vi "Default Cfg File Path.vi"(8 "error in (no error)":errorcluster) -> (0 "error out":errorcluster, 3 "Default Path":path)   [LabVIEW 2018]
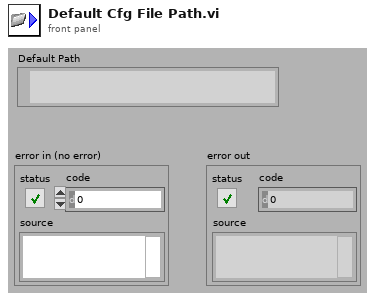
[diagram p1: front panel]
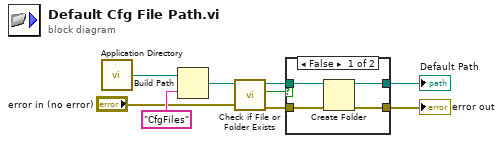
[diagram p0: block diagram]
diagram:
  n1 = call <vilib>:"Application Directory.vi"() -> ("Application Directory"=w8:path)
  n2 = Build Path(base path=w8, name or relative path="CfgFiles") -> (appended path=w4:path)
  n3 = call <vilib>:"Check if File or Folder Exists.vi"("error in (no error)"="error in (no error)", "path"=w4) -> ("error out"=w5:errorcluster, "file or folder exists?"=w6:bool, "dup path"=w7:path)  [unwired: 7 in]
  n4 = case shown="False" w6 {
    tunnel: w7 -> [w13 w14]
    tunnel: w5 -> [w12 w15]
    tunnel: [w11 w15] -> w2
    tunnel: [w10 w14] -> w3
    frame False {
      n5 = Create Folder(path (use dialog)=w13, error in=w12) -> (created path=w10:path, error out=w11:errorcluster)  [unwired: 1 in, 1 out]
    }
    frame True {
    }
  }
  "Default Path" <- w3
  "error out" <- w2
